vi "Read TEC Enable.vi"(8 "error in (no error)":errorcluster, 11 "Set TEC Enable MSG in":refnum<class "Set TEC Enable MSG.lvclass">) -> (0 "error out":errorcluster, 2 "TEC Enable":bool[](array[boolean]), 3 "Set TEC Enable MSG out":refnum<class "Set TEC Enable MSG.lvclass">)   [LabVIEW 2014, in "Set TEC Enable MSG.lvclass"]
uses:
  Set TEC Enable MSG.lvclass
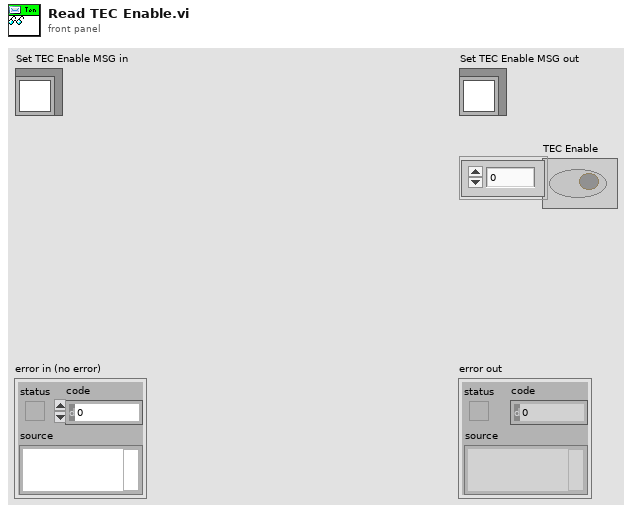
[diagram p1: front panel]
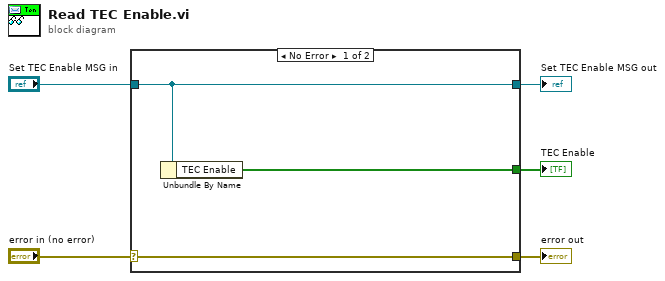
[diagram p0: block diagram]
diagram:
  n1 = case shown="No Error" "error in (no error)" {
    selector: "error in (no error)" -> [w8 w9]
    tunnel: [w8 w9] -> w4
    tunnel: [w7 w10] -> w2
    tunnel: "Set TEC Enable MSG in" -> [w7 w10]
    tunnel: [w6 _] -> w1
    frame No Error {
      n2 = Unbundle By Name(w7) -> ("TEC Enable"=w6:bool[])
    }
    frame Error {
    }
  }
  "error out" <- w4
  "Set TEC Enable MSG out" <- w2
  "TEC Enable" <- w1
